vi "Webmessages.vi"() -> ()   [LabVIEW 2024]
uses:
  <vilib>/sklein/WebView2/Webview2 Control/WebView2 Control.xctl
panel:
  in  "Background":u32(colorbox)
  in  "stop":bool
  in  "Set JS":bool
  in  "Msg":bool
  out "Message from Page":string
  in  "Message to Page":string
  out "WebView2 Control":string(xcontrol)
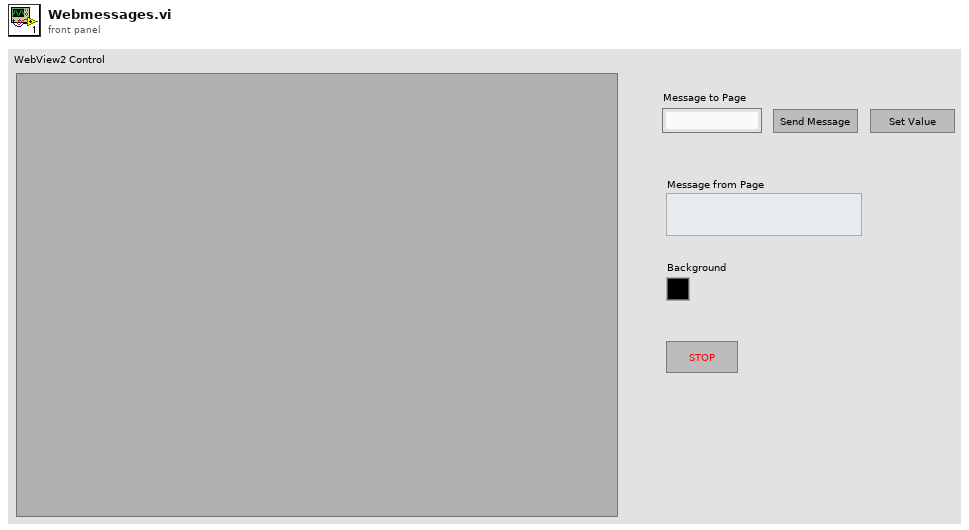
[diagram p1: front panel]
types:
  T1 = typedef "WebView2 Control.xctl/Events.ctl" = cluster{"Navigation Complete Event":refnum<user-event>, "Source Changed Event":refnum<user-event>, "Document Title Changed Event":refnum<user-event>, "Status Bar Text Changed":refnum<user-event>, "Web Message Received":refnum<user-event>, "Window Close Requested":refnum<user-event>, "DOM Loaded":refnum<user-event>, "Navigation Started Event":refnum<user-event>}
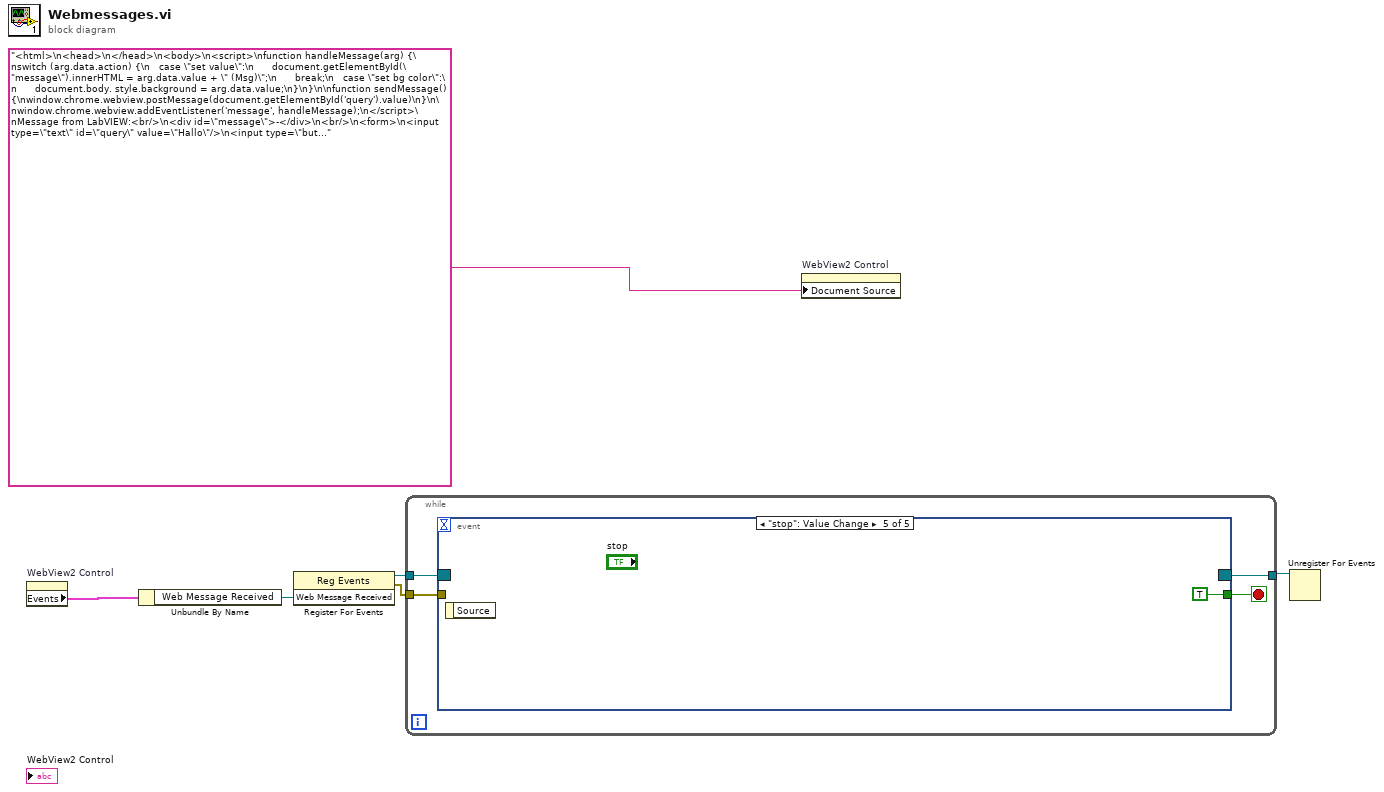
[diagram p0: block diagram]
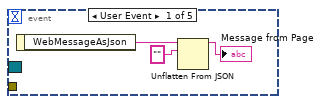
[diagram p2: hidden frame]
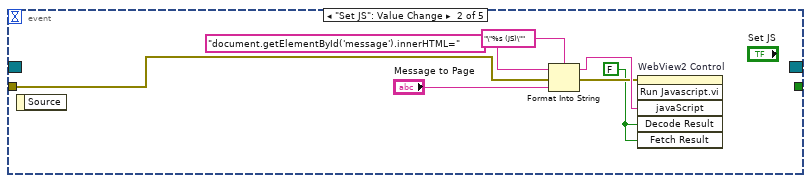
[diagram p3: hidden frame]
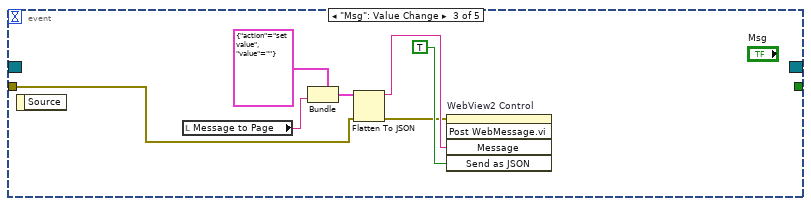
[diagram p4: hidden frame]
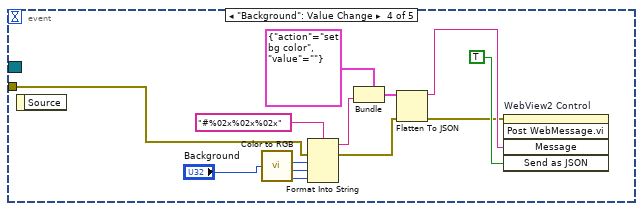
[diagram p5: hidden frame]
diagram:
  n1 = property on="WebView2 Control" class="WebView2 Control (strict)"() -> ("Events"=w5:T1)  [unwired: 2 in, 2 out]
  n2 = Unbundle By Name(w5) -> ("Web Message Received"=w2:refnum<user-event>)
  n3 = register-events(w2) -> (reference out=w4:refnum<event-registration>, error out=w3:errorcluster)  [unwired: 2 in]
  n4 = while {
    tunnel: w4 -> [w8]
    tunnel: w3 -> [w9]
    tunnel: [w7] -> w1
    stop <- w10 stop-if-true
    n5 = event shown="[4] \"stop\": Value Change" {
      selector: w8 -> [_ _ _ _ _]
      dyn-events: [_ _ _ _ _] -> w7
      timeout: _ -> [_ _ _ _ _]
      tunnel: [_ _ _ _ TRUE] -> w10
      tunnel: w9 -> [_ w15 w22 w28 _]
      event User Event {
        n6 = event-data() -> ("WebMessageAsJson"=w13:string)  [unwired: 1 in]
        n7 = Unflatten From JSON(JSON string=w13, type and defaults="") -> (value=→"Message from Page":string)  [unwired: 5 in, 1 out]
      }
      event "Set JS": Value Change {
        w14 = FALSE ("Fetch Result")
        n8 = event-data() -> ()  [unwired: 1 in, 1 out]
        n9 = Format Into String(format string="\"%s (JS)\"", initial string="document.getElementById('message').innerHTML=" ("javaScript"), error in=w15, "Message to Page") -> (resulting string=w19:string, error out=w16:errorcluster)
        n10 = invoke on="WebView2 Control" class="WebView2 Control (strict)" method="Run Javascript.vi"(error in=w16, "javaScript"=w19, "Decode Result"=w14, "Fetch Result"=w14) -> ()  [unwired: 2 in, 6 out]
      }
      event "Msg": Value Change {
        n11 = event-data() -> ()  [unwired: 1 in, 1 out]
        n12 = local read "Message to Page"() -> (w23:string)
        n13 = Bundle(cluster=cluster{"action":string, "value":string} {"action"="set value", "value"=""}, "value"=w23) -> (w26:cluster{"action":string, "value":string})  [unwired: 1 in]
        n14 = Flatten To JSON(anything=w26, error in (no error)=w22) -> (JSON string=w25:string, 11:w21:errorcluster)  [unwired: 1 in]
        n15 = invoke on="WebView2 Control" class="WebView2 Control (strict)" method="Post WebMessage.vi"(error in=w21, "Message"=w25, "Send as JSON"=TRUE) -> ()  [unwired: 2 in, 5 out]
      }
      event "Background": Value Change {
        n16 = event-data() -> ()  [unwired: 1 in, 1 out]
        n17 = call <vilib>:"Color to RGB.vi"("Color"="Background") -> ("R"=w32:u8, "G"=w31:u8, "B"=w30:u8)  [unwired: 1 out]
        n18 = Format Into String(format string="#%02x%02x%02x", error in=w28, w32, w31, w30) -> (resulting string=w35:string, error out=w34:errorcluster)  [unwired: 1 in]
        n19 = Bundle(cluster=cluster{"action":string, "value":string} {"action"="set bg color", "value"=""}, "value"=w35) -> (w39:cluster{"action":string, "value":string})  [unwired: 1 in]
        n20 = Flatten To JSON(anything=w39, error in (no error)=w34) -> (JSON string=w38:string, 11:w29:errorcluster)  [unwired: 1 in]
        n21 = invoke on="WebView2 Control" class="WebView2 Control (strict)" method="Post WebMessage.vi"(error in=w29, "Message"=w38, "Send as JSON"=TRUE) -> ()  [unwired: 2 in, 5 out]
      }
      event "stop": Value Change {
        n22 = event-data() -> ()  [unwired: 1 in, 1 out]
      }
    }
  }
  n23 = property on="WebView2 Control" class="WebView2 Control (strict)"("Document Source"="<html>\n<head>\n</head>\n<body>\n<script>\nfunction handleMessage(arg) {\nswitch (arg.data.action) {\n   case \"set value\":\n      document.getElementById(\"message\").innerHTML = arg.data.value + \" (Msg)\";\n      break;\n   case \"set bg color\":\n      document.body. style.background = arg.data.value;\n}\n}\n\nfunction sendMessage() {\nwindow.chrome.webview.postMessage(document.getElementById('query').value)\n}\n\nwindow.chrome.webview.addEventListener('message', handleMessage);\n</script>\nMessage from LabVIEW:<br/>\n<div id=\"message\">-</div>\n<br/>\n<form>\n<input type=\"text\" id=\"query\" value=\"Hallo\"/>\n<input type=\"button\" onclick=\"sendMessage()\" value=\"Send To LabVIEW\">\n</body>\n</html>") -> ()  [unwired: 2 in, 2 out]
  n24 = Unregister For Events(event registration refnum=w1) -> ()  [unwired: 1 in, 1 out]
